vi "TW Replace Missing Dependency VIs - Client Wrapper.vi"(8 "error in":errorcluster, 10 "gRPC Service Name":string, 11 "Template Project Path":path) -> (0 "error out":errorcluster)   [LabVIEW 2021, in "Plugin Generator.lvlib"]
uses:
  Plugin Generator.lvlib
  <vilib>/CIF Foundation/CIF LabVIEW Scripting/LV Scripting/LV Scripting Utilities.lvlib
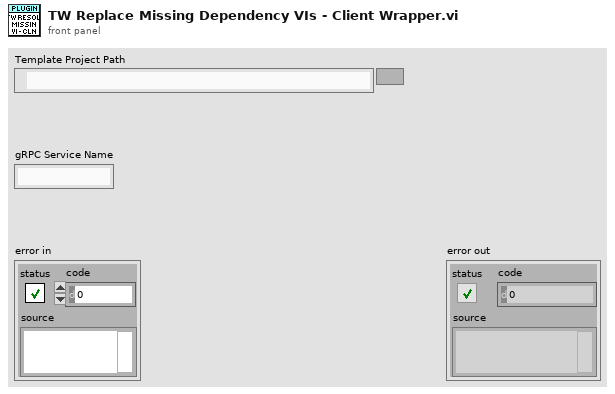
[diagram p1: front panel]
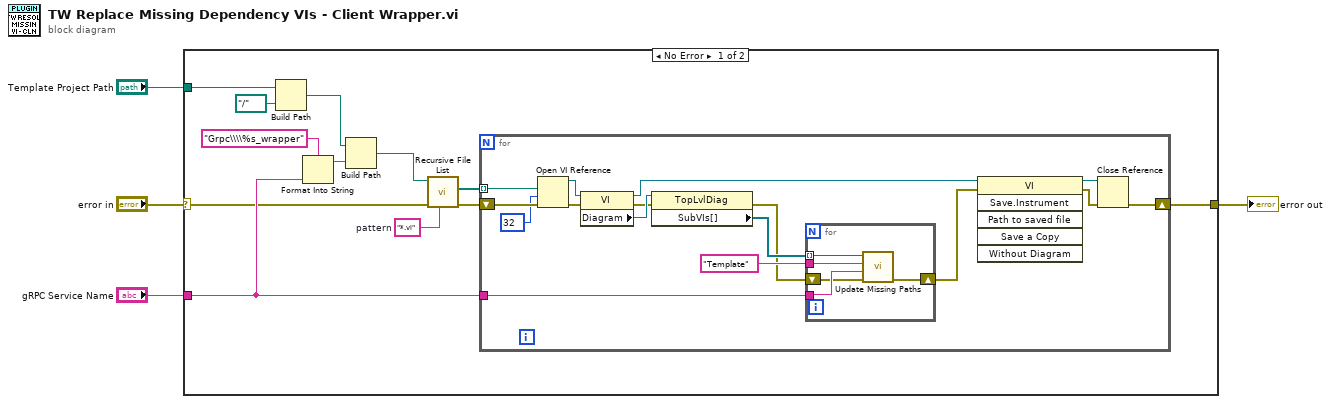
[diagram p0: block diagram]
diagram:
  n1 = case shown="No Error" "error in" {
    selector: "error in" -> [w9 w38]
    tunnel: [w8 w38] -> w4
    tunnel: "gRPC Service Name" -> [w11 _]
    tunnel: "Template Project Path" -> [w6 _]
    frame No Error {
      w15 = "*.vi"  # pattern
      n2 = Build Path(base path=w6, name or relative path=path "../..") -> (appended path=w5:path)
      n3 = Format Into String(format string="Grpc\\\\%s_wrapper" ("Class Name"), w11) -> (resulting string=w14:string)  [unwired: 2 in, 1 out]
      n4 = Build Path(base path=w5, name or relative path=w14) -> (appended path=w13:path)
      n5 = call <vilib>:"Recursive File List.vi"("pattern"=w15, "error in (no error)"=w9, "Folder Path"=w13) -> ("error out"=w10:errorcluster, "All Files in Dir"=w16:path[])  [unwired: 4 in, 3 out]
      n6 = for {
        tunnel: w16 -> [w32] mode=indexing
        tunnel: w11 -> [w31]
        shift-right: [w30] -> w8
        shift-left: w10 -> [w29]
        n7 = Open VI Reference(vi path=w32, options=32, error in (no error)=w29) -> (vi reference=w28:refnum<vi>, error out=w23:errorcluster)  [unwired: 3 in]
        n8 = property class="VI"(reference=w28, error in=w23) -> (reference out=w26:refnum<vi>, error out=w24:errorcluster, "Diagram"=w27:refnum<vi>)
        n9 = property class="TopLvlDiag"(reference=w27, error in=w24) -> (error out=w18:errorcluster, "SubVIs[]"=w25:refnum<vi>[])  [unwired: 1 out]
        n10 = for {
          tunnel: w25 -> [w37] mode=indexing
          tunnel: w31 -> [w34]
          tunnel: "Template" ("search string") -> [w35]
          shift-right: [w36] -> w17
          shift-left: w18 -> [w33]
          n11 = call <vilib>:"Update Missing Paths.vi"("error in (no error)"=w33, "New Subname"=w34, "Subname to Replace"=w35, "GObject in"=w37) -> ("error out"=w36:errorcluster)  [unwired: 7 in]
        }
        n12 = invoke class="VI" method="Save.Instrument"(reference=w26, error in=w17) -> (reference out=w21:refnum<vi>, error out=w20:errorcluster)  [unwired: 4 in, 4 out]
        n13 = Close Reference(reference=w21, error in (no error)=w20) -> (error out=w30:errorcluster)
      }
    }
    frame Error {
    }
  }
  "error out" <- w4
